vi "DriveToDistance.vi"(8 "Error In":errorcluster, 10 "Setpoint":dbl) -> (0 "Error Out":errorcluster)   [LabVIEW 2016]
uses:
  <vilib>/Rock Robotics/WPI/Ultrasonic/WPI_SonarMB1010AnalogRefNum Registry Get.vi
  <vilib>/Rock Robotics/WPI/Ultrasonic/WPI_SonarMB1010AnalogGetRange.vi
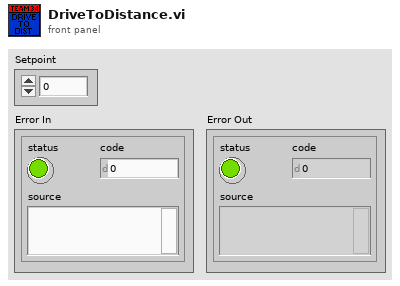
[diagram p1: front panel]
types:
  T1 = typedef "WPI_SonarMB1010AnalogDeviceRef.ctl" = cluster{"AIDeviceRef":T2, "Scaling factor (V/in)":dbl, "Average Bits":u8}
  T2 = typedef "WPI_AnalogChannelDevRef.ctl" = cluster{"DevStatus":errorcluster, "Analog Channel":T3}
  T3 = typedef "FPGA_AIChannel.ctl" = enum8{"AI 0", "AI 1", "AI 2", "AI 3", "AI MXP 0", "AI MXP 1", "AI MXP 2", "AI MXP 3", "Invalid"}
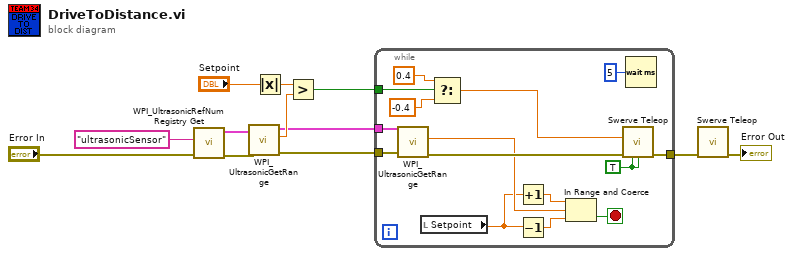
[diagram p0: block diagram]
diagram:
  n1 = call-poly <vilib>:"WPI_UltrasonicRefNum Registry Get.vi"("error in (no error)"="Error In", "refnum name"="ultrasonicSensor") -> ("error out"=w8:errorcluster, "SonarMB1010AnalogDevRef"=w6:T1)  [unwired: 8 in]
  n2 = call-poly <vilib>:"WPI_UltrasonicGetRange.vi"("error in"=w8, "SonarMB1010AnalogDevRef"=w6) -> ("error out"=w9:errorcluster, "Distance"=w10:dbl, "SonarMB1010AnalogDevRef"=w7:T1)  [unwired: 7 in]
  n3 = Absolute Value(x="Setpoint") -> (abs(x)=w11:dbl)
  n4 = Greater?(x=w11, y=w10) -> (0:w12:bool)
  n5 = while {
    tunnel: [w27] -> w5
    tunnel: w7 -> [w26]
    tunnel: w9 -> [w25]
    tunnel: w12 -> [w22]
    stop <- w17 stop-if-true
    w23 = TRUE ("Robot Centric?")
    n6 = call-poly <vilib>:"WPI_UltrasonicGetRange.vi"("error in"=w25, "SonarMB1010AnalogDevRef"=w26) -> ("error out"=w24:errorcluster, "Distance"=w18:dbl)  [unwired: 7 in, 1 out]
    n7 = local read "Setpoint"() -> (w13:dbl)
    n8 = Select(t=0.4, s=w22, f=-0.4) -> (s? t:f=w15:dbl)
    n9 = Increment(x=w13) -> (x+1=w20:dbl)
    n10 = Decrement(x=w13) -> (x-1=w19:dbl)
    n11 = In Range and Coerce(upper limit=w20, x=w18, lower limit=w19) -> (In Range?=w17:bool)  [unwired: 1 out]
    n12 = call "Swerve Teleop.vi"("Y"=w15, "Error In"=w24, "Robot Centric?"=w23, "Autonomous?"=w23) -> ("Error Out"=w27:errorcluster)  [unwired: 7 in, 4 out]
    n13 = Wait (ms)(milliseconds to wait=u32 5) -> ()  [unwired: 1 out]
  }
  n14 = call "Swerve Teleop.vi"("Error In"=w5) -> ("Error Out"=→"Error Out":errorcluster)  [unwired: 10 in, 4 out]
